vi "Gap7b.vi"(11 "GIC Input":T2={"     Use ?\nOff       On"=[FALSE, TRUE, FALSE, TRUE], "Mode:"=FALSE, "Extra Port"="", "Hokuyo Port"="COM7", "Tx Prop  Port"="COM6", "Compass Port"="", "GPS Port"="", "Num of WPs"=0, "WP Lats and Longs"={"WP Lats"=[], "WP Longs"=[]}, "Obst Lats and Longs"={"Obst Lats"=[], "Obst Longs"=[]}, "Parameters"=[], "GPS Data"=[], "Compass"=0.0, "LMS Vector"=[], "Vision Vector"=[], "Direction Cmd"=0.0, "Speed Cmd"=0.0, "WP Vector"=[], "WP Number"=0, "Extra"=0, "SW Map"=[], "Path Cluster"={"Path x node"=[], "Path y node"=[]}, "Sim Course"=[]} {"Obst Lats and Longs"."Obst Longs" format="%#_8g"; "Obst Lats and Longs"."Obst Lats" format="%#_8g"}) -> (3 "GIC Output":T1={"     Use ?\nOff       On"=[FALSE, TRUE, FALSE, TRUE], "Mode:"=FALSE, "Extra Port"="", "Hokuyo Port"="COM7", "Tx Prop Port"="COM6", "Compass Port"="", "GPS Port"="", "Num of WPs"=0, "WP Lats and Longs"={"WP Lats"=[], "WP Longs"=[]}, "Obst Lats and Longs"={"Obst Lats"=[], "Obst Longs"=[]}, "Parameters"=[], "GPS Data"=[], "Compass"=0.0, "LMS Vector"=[], "Vision Vector"=[], "Direction Cmd"=0.0, "Speed Cmd"=0.0, "WP Vector"=[], "WP Number"=0, "Extra"=0, "SW Map"=[], "Path Cluster"={"Path x node"=[], "Path y node"=[]}, "Sim Course"=[]} {"Obst Lats and Longs"."Obst Longs" format="%#_8g"; "Obst Lats and Longs"."Obst Lats" format="%#_8g"})   [LabVIEW 2014]
panel:
  out "ya":dbl
  out "xa":dbl
  out "dl23":dbl
  out "dr23":dbl
  out "a":dbl
  out "s":dbl
  out "objy":dbl
  out "objx":dbl
  out "dl":dbl
  out "dr":dbl
  out "dl45":dbl
  out "dr45":dbl
  out "d0":dbl
  # "GAP 7B Program\nSpeed is verticle"
  # "Input:"
  # "Output"
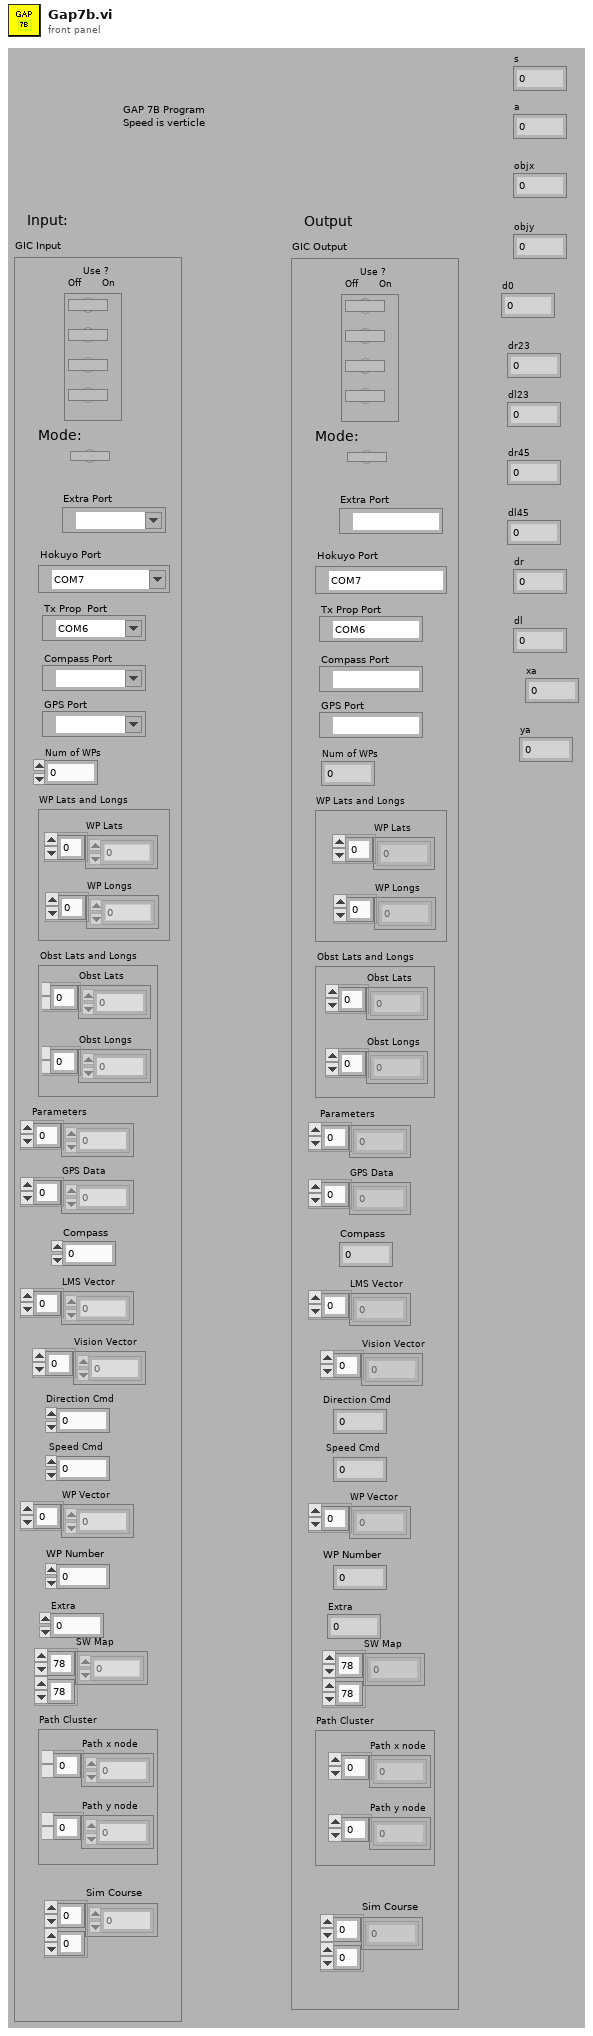
[diagram p1: front panel]
types:
  T1 = cluster{"     Use ?\nOff       On":bool[], "Mode:":bool, "Extra Port":refnum<visa-resource-name>, "Hokuyo Port":refnum<visa-resource-name>, "Tx Prop Port":refnum<visa-resource-name>, "Compass Port":refnum<visa-resource-name>, "GPS Port":refnum<visa-resource-name>, "Num of WPs":i16, "WP Lats and Longs":cluster{"WP Lats":dbl[], "WP Longs":dbl[]}, "Obst Lats and Longs":cluster{"Obst Lats":dbl[], "Obst Longs":dbl[]}, "Parameters":dbl[], "GPS Data":dbl[], "Compass":dbl, "LMS Vector":dbl[], "Vision Vector":dbl[], "Direction Cmd":dbl, "Speed Cmd":dbl, "WP Vector":dbl[], "WP Number":i32, "Extra":i16, "SW Map":i32[][], "Path Cluster":cluster{"Path x node":dbl[], "Path y node":dbl[]}, "Sim Course":i8[][]}
  T2 = cluster{"     Use ?\nOff       On":bool[], "Mode:":bool, "Extra Port":refnum<visa-resource-name>, "Hokuyo Port":refnum<visa-resource-name>, "Tx Prop  Port":refnum<visa-resource-name>, "Compass Port":refnum<visa-resource-name>, "GPS Port":refnum<visa-resource-name>, "Num of WPs":i16, "WP Lats and Longs":cluster{"WP Lats":dbl[], "WP Longs":dbl[]}, "Obst Lats and Longs":cluster{"Obst Lats":dbl[], "Obst Longs":dbl[]}, "Parameters":dbl[], "GPS Data":dbl[], "Compass":dbl, "LMS Vector":dbl[], "Vision Vector":dbl[], "Direction Cmd":dbl, "Speed Cmd":dbl, "WP Vector":dbl[], "WP Number":i32, "Extra":i16, "SW Map":i32[][], "Path Cluster":cluster{"Path x node":dbl[], "Path y node":dbl[]}, "Sim Course":i8[][]}
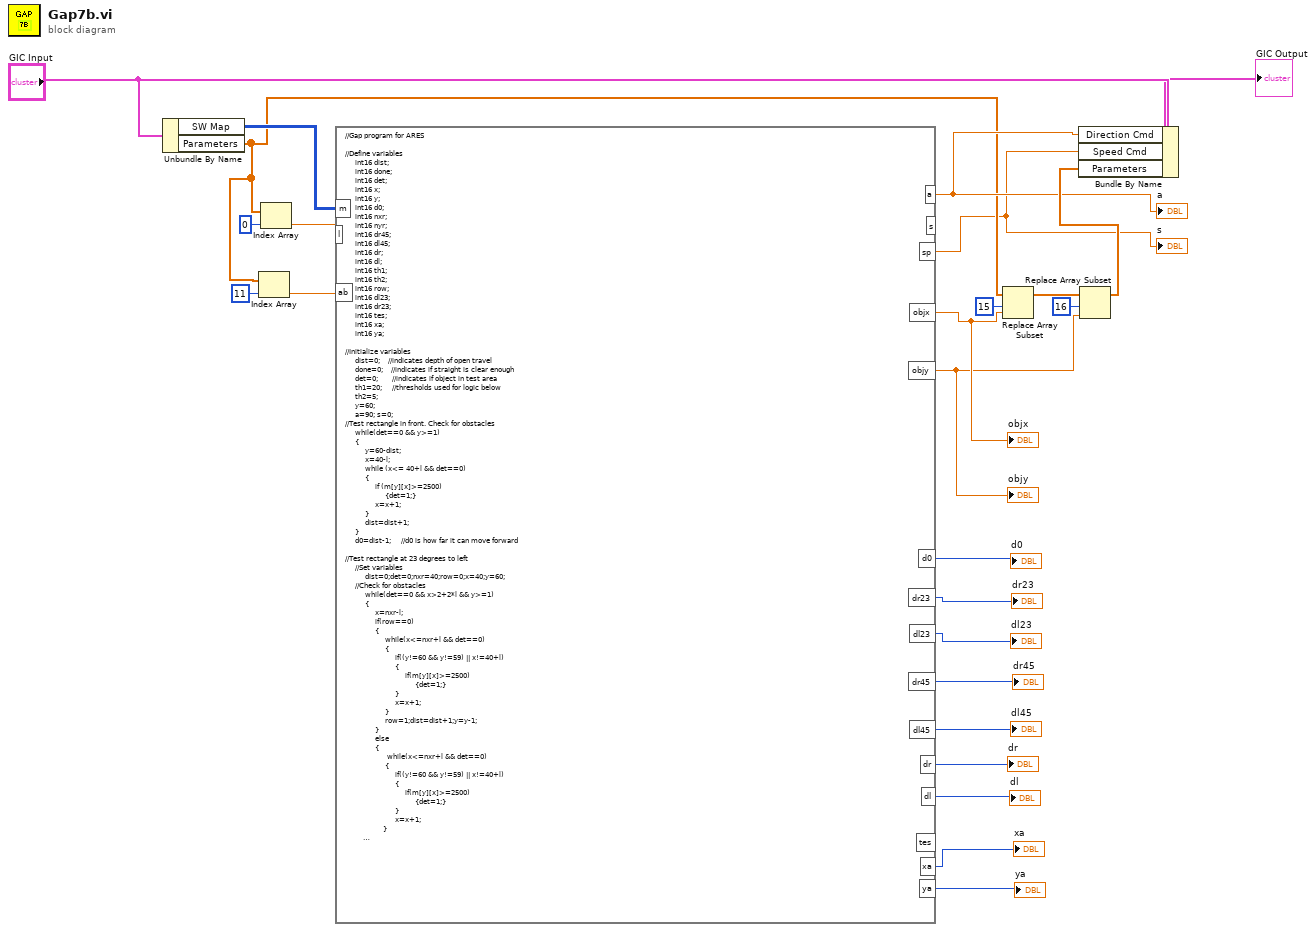
[diagram p0: block diagram]
diagram:
  n1 = Unbundle By Name("GIC Input") -> ("SW Map"=w25:i32[][], "Parameters"=w6:dbl[])
  n2 = Index Array(array=w6, index=11) -> (element=w4:dbl)
  n3 = Index Array(array=w6, index=0) -> (element=w23:dbl)
  n4 = formula code="//Gap program for ARES\n\n//Define variables\n     int16 dist;\n     int16 done;\n     int16 det;\n     int16 x;\n     int16 y;\n     int16 d0;\n     int16 nxr;\n     int16 nyr;\n     int16 dr45;\n     int16 dl45;\n     int16 dr;\n     int16 dl;\n     int16 th1;\n     int16 th2;\n     int16 row;\n     int16 dl23;\n     int16 dr23;\n     int16 tes;\n     int16 xa;\n     int16 ya;\n\n//Initialize variables\n     dist=0;    //indicates depth of open travel\n     done=0;    //indicates if straight is clear enough\n     det=0;       //indicates if object in test area\n     th1=20;     //thresholds used for logic below\n     th2=5;\n     y=60;\n     a=90; s=0;\n//Test rectangle in front. Check for obstacles\n     while(det==0 && y>=1)\n     {\n          y=60-dist;\n          x=40-l;\n          while (x<= 40+l && det==0)\n          {\n               if (m[y][x]>=2500)\n                    {det=1;}\n               x=x+1;\n          }\n          dist=dist+1;\n     }\n     d0=dist-1;     //d0 is how far it can move forward\n\n//Test rectangle at 23 degrees to left\n     //Set variables\n          dist=0;det=0;nxr=40;row=0;x=40;y=60;\n     //Check for obstacles\n          while(det==0 && x>2+2*l && y>=1)\n          {\n               x=nxr-l;\n               if(row==0)\n               {\n                    while(x<=nxr+l && det==0)\n                    {\n                         if((y!=60 && y!=59) || x!=40+l)\n                         {\n                              if(m[y][x]>=2500)\n                                   {det=1;}\n                         }\n                         x=x+1;\n                    }\n                    row=1;dist=dist+1;y=y-1;\n               }\n               else\n               {\n                     while(x<=nxr+l && det==0)\n                    {\n                         if((y!=60 && y!=59) || x!=40+l)\n                         {\n                              if(m[y][x]>=2500)\n                                   {det=1;}\n                         } \n                         x=x+1;\n                   }\n                    row=0;dist=dist+1;y=y-1; nxr=nxr-1;\n              }  \n          }  \n          dl23=dist-1;  \n\n//Test rectangle at 23 degrees to right\n     //Set variables\n          dist=0;det=0;nxr=40;row=0;x=40;y=60;\n     //Check for obstacles\n          while(det==0 && x<=77 && y>=1)\n          {\n               x=nxr-l;\n               if(row==0)\n               {\n                    while(x<=nxr+l && det==0)\n                    {\n                         if((y!=60 && y!=59) || x!=40-l)\n                         {\n                              if(m[y][x]>=2500)\n                                   {det=1;}\n                         }\n                         x=x+1;\n                    }\n                    row=1;dist=dist+1;y=y-1;\n               }\n               else\n               {\n                      while(x<=nxr+l && det==0)\n                    {\n                         if((y!=60 && y!=59) || x!=40-l)\n                         {\n                              if(m[y][x]>=2500)\n                                   {det=1;}\n                         }\n                         x=x+1;\n                    }\n                    row=0;dist=dist+1;y=y-1; nxr=nxr+1;\n               }\n          }\n          dr23=dist-1;   \n\n//If room to the front or 23 degree to either side, just go there\n     //if(d0>=th1 || dr23>=th1 || dl23>=th1)\n          //{done=1;}\n\n//Test rectangle at 45 degrees to right\n     //Set variables\n          dist=0;det=0;nxr=40;nyr=60;x=40;\n     //Check for obstacles\n          while(det==0 && x<=77)\n          {\n               x=nxr-l; y=nyr-l;\n               while(x<=nxr+l && det==0)\n                    {\n                         if(m[y][x]>=2500)\n                              {det=1;}\n                         if(m[y-1][x]>=2500)\n                              {det=1;}\n                         if(x==nxr+l)\n                         {\n                              if(m[y][x+1]>=2500)\n                                   {det=1;}\n                         }\n                         x=x+1; y=y+1;\n                    }\n                    nxr=nxr+1;nyr=nyr-1;\n                    dist=dist+1;\n          }\n          dr45=dist-1;\n\n//Test rectangle at 45 degrees to left\n     //Set variables\n          dist=0;det=0;nxr=40;nyr=60;x=40;\n     //Check for obstacles\n          while(det==0 && x>=2+2*l)\n          {\n               x=nxr-l; y=nyr+l;\n               while(x<=nxr+l && det==0)\n                    {\n                         if(m[y][x]>=2500)\n                              {det=1;}\n                         if(m[y][x-1]>=2500)\n                              {det=1;}\n                         if(x==nxr+l)\n                         {\n                              if(m[y-1][x]>=2500)\n                                   {det=1;}\n                         }\n                         x=x+1; y=y-1;\n                    }\n                    nxr=nxr-1;nyr=nyr-1;\n                    dist=dist+1;\n          }\n          dl45=dist-1;   \n\n//Test rectangle to the right (right below and above robot)\n     //Set variables\n          dist=0;det=0; x=0;\n          while(det==0 && x<=78)\n          {\n               x=40+dist; y=60+l;\n               while(y>=60-l && det==0)\n               {\n                    if (m[y][x] >=2500)\n                         {det=1;}\n                    y=y-1;\n               }\n               dist=dist+1;\n          }\n          dr=dist-1;\n\n//Test rectangle to the left (left below and above robot)\n     //Set variables\n          dist=0;det=0; x=1;\n          while(det==0 && x>=1)\n          {\n               x=40-dist; y=60+l;\n               while(y>=60-l && det==0)\n               {\n                    if (m[y][x] >=2500)\n                         {det=1;}\n                    y=y-1;\n               }\n               dist=dist+1;\n          }\n          dl=dist-1;\n\n//Go in direction of longest distance at speed proportional to distance\n\n          if(d0>th2 || dr45 >th2 || dl45>th2 || dr>th2 || dl>th2 || dr23>th2 || dl23>th2)\n          {\n               if(d0>=dr45 && d0>=dl45 && d0>=dr && d0>=dl && d0>=dr23 && d0>= dl23)\n                    {s=d0;a=90 + (dl23 - dr23)/3;}\n               if(dr45>d0 && dr45>=dl45 && dr45>=dr && dr45>=dl && dr45>dr23 && dr45>dl23)\n                    {s=dr45;a=45;}\n               if(dl45>d0 && dl45>dr45 && dl45 >=dr && dl45>=dl && dl45>dr23 && dl45>dl23)\n                    {s=dl45;a=135;}\n               if(dr>d0 && dr>dr45 && dr>dl45 && dr>=dl && dr>dr23 && dr>dl23)\n                    {s=dr;a=0;}\n                if(dl>d0 && dl>dr45 && dl>dl45 && dl>dr && dl>dr23 && dl>dl23)\n                    {s=dl;a=180;}\n                if(dr23>d0 && dr23>=dl23 && dr23>=dr45 && dr23>=dl45 && dr23>=dr && dr23>=dl)\n                    {s=dr23;a=67 + (d0 - dr45)/3;}\n                if(dl23>d0 && dl23>dr23 && dl23>=dr45 && dl23>=dl45 && dl23>=dr && dl23>=dl)\n                    {s=dl23;a=113 + (dl45 - d0)/3;}\n                 objx=40+cos(a*0.017453)*s;\n                 objy=60-sin(a*0.017453)*s;\n          }\n          else\n          {s=30;a=270; objx=40; objy = 79;}\n     \n//Make speed command only the verticle component for sabertooth mixed mode\n     sp = (71* abs(objy - 60))/60;\n\n//Angle bias\n     a=a+ab;"("m"=w25, "l"=w23, "ab"=w4) -> ("a"=w11:dbl, "objx"=w13:dbl, "objy"=w12:dbl, "d0"=→"d0":i16, "dr45"=→"dr45":i16, "dl45"=→"dl45":i16, "dr"=→"dr":i16, "dl"=→"dl":i16, "dr23"=→"dr23":i16, "dl23"=→"dl23":i16, "xa"=→"xa":i16, "ya"=→"ya":i16, "sp"=w1:dbl)  [unwired: 2 out]
  "objx" <- w13
  "objy" <- w12
  "s" <- w1
  "a" <- w11
  n5 = Replace Array Subset(array=w6, new element=w13, index=15) -> (w21:dbl[])
  n6 = Replace Array Subset(array=w21, new element=w12, index=16) -> (w19:dbl[])
  n7 = Bundle By Name(cluster="GIC Input", "Direction Cmd"=w11, "Speed Cmd"=w1, "Parameters"=w19) -> (→"GIC Output":T2)
